vi "programTSLAspic2.vi"(8 "clock manuelle":bool, 9 "clockdata 2":u32[](array[numeric])=[65535, 65535, 65535, 65535, 65535, 65535, 65535, 65535, 65535, 65535, 65535, 65535, 65535, 65535, 65535, 65535, 0, 2147483648, 0, 2147483648, 0, 2147483648, 0, 2147483648, 0, 2147483648, 0, 2147483648, 0, 2147483648, 0, 2147483648, 0] format="%08x", 10 "repetitions":u32=1048575 format="%08x", 11 "pathTSFile":path=path "C:/damic/DAMIC_TIMESLICE/DamicDebugADC18test2.txt" caption="Path to timeslice file") -> (1 "outputClockData":u32[](array[numeric]), 2 "error out 2":errorcluster)   [LabVIEW 2014]
uses:
  <vilib>/Utility/file.llb/Read From Spreadsheet File (I64).vi
panel:
  out "String":string
  in  "clockmessagetype":u32=286331153 format="%x"
  in  "clockdata":u32[](array[numeric])=[65535, 65535, 65535, 65535, 65535, 65535, 65535, 65535, 65535, 65535, 65535, 65535, 65535, 65535, 65535, 65535, 0, 2147483648, 0, 2147483648, 0, 2147483648, 0, 2147483648, 0, 2147483648, 0, 2147483648, 0, 2147483648, 0, 2147483648, 0] format="%08x"
  in  "clockitems":u8=33
  out "resolution (ns)":u32
  out "number of signals":u32
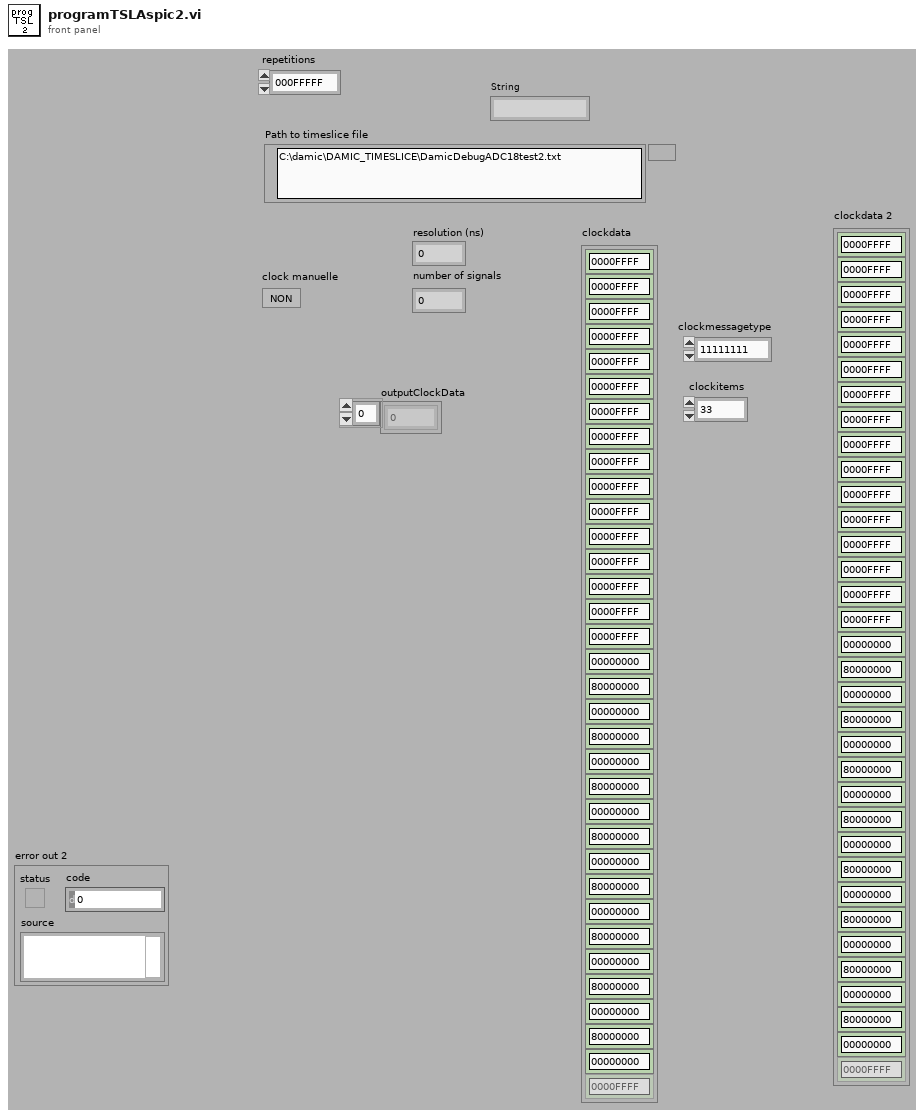
[diagram p1: front panel]
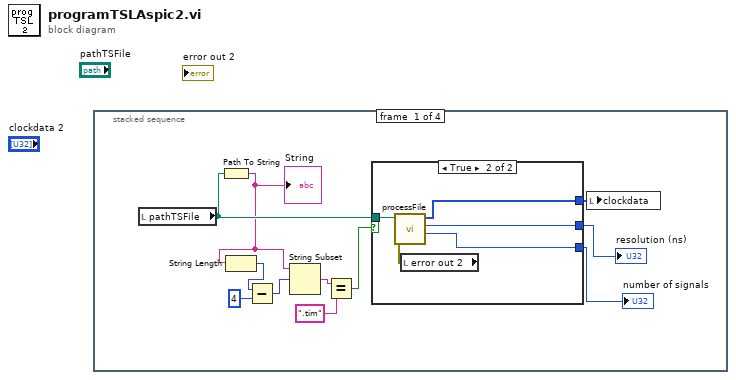
[diagram p0: block diagram]
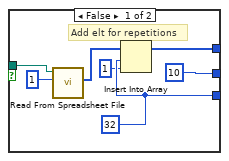
[diagram p2: hidden frame]
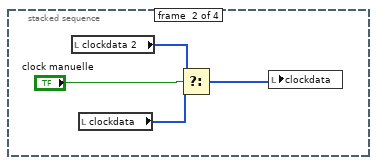
[diagram p3: hidden frame]
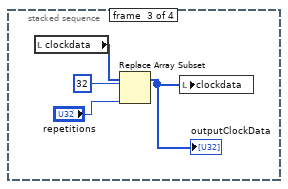
[diagram p4: hidden frame]
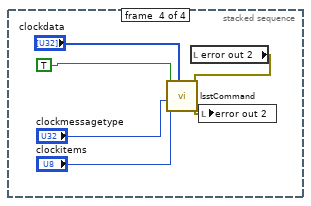
[diagram p5: hidden frame]
diagram:
  n1 = stacked-sequence {
    frame #0 {
      n2 = local read "pathTSFile"() -> (w8:path)
      n3 = Path To String(path=w8) -> (string=w1:string)
      "String" <- w1
      n4 = String Length(string=w1) -> (length=w7:i32)
      n5 = Subtract(x=w7, y=4) -> (x-y=w5:i32)
      n6 = String Subset(string=w1, offset (0)=w5) -> (substring=w4:string)  [unwired: 1 out]
      n7 = Equal?(x=w4, y=".tim") -> (x = y?=w2:bool)
      n8 = case shown="True" w2 {
        tunnel: [w14 w22] -> w11
        tunnel: [w13 w21] -> w10
        tunnel: [u32 10 ("resolution") w20] -> w9
        tunnel: w8 -> [w18 w19]
        frame False {
          w13 = u32 32 ("numberSignals")
          # "Add elt for repetitions"
          n9 = call-poly <vilib>:"Read From Spreadsheet File.vi"("number of rows (all:-1)"=1, "file path (dialog if empty)"=w18) -> ("first row"=w17:i64[])  [unwired: 2 in, 7 out]
          n10 = Insert Into Array(array=w17, index=w13, new element=i64 1 ("new element/subarray")) -> (w14:i64[])
        }
        frame True {
          n11 = local read "error out 2"() -> (w23:errorcluster)
          n12 = call "processFile.vi"("error in"=w23, "selected path"=w19) -> ("numberSignals"=w21:u32, "resolution"=w20:u32, "readyData"=w22:u32[])  [unwired: 6 out]
        }
      }
      "resolution (ns)" <- w9
      "number of signals" <- w10
      n13 = local write "clockdata"(w11) -> ()
    }
    frame #1 {
      n14 = local read "clockdata 2"() -> (w27:u32[])
      n15 = local read "clockdata"() -> (w26:u32[])
      n16 = Select(t=w27, s="clock manuelle", f=w26) -> (s? t:f=w25:u32[])
      n17 = local write "clockdata"(w25) -> ()
    }
    frame #2 {
      n18 = local read "clockdata"() -> (w31:u32[])
      n19 = Replace Array Subset(array=w31, new element="repetitions", index=32) -> (w28:u32[])
      "outputClockData" <- w28
      n20 = local write "clockdata"(w28) -> ()
    }
    frame #3 {
      n21 = local read "error out 2"() -> (w33:errorcluster)
      n22 = call "lsstCommand.vi"("error in (no error)"=w33, "data"="clockdata", "nbitems"="clockitems", "messagetype"="clockmessagetype", "execute"=TRUE) -> ("error out"=w32:errorcluster)  [unwired: 2 in, 4 out]
      n23 = local write "error out 2"(w32) -> ()
    }
  }
